vi "Send Receive Parse.vi"(8 "error in":errorcluster, 10 "Delay between send and receive [ms]":i32=100, 11 "<JSON>":string="{  \n    \"command\": \"ccd_discover\",\n    \"parameters\":{\n        \"index\": 0\n    }\n}") -> (0 "error out":errorcluster, 2 "ID":i32, 3 "results-JSON string":string)   [LabVIEW 2023, in "GenericDevice.lvclass"]
doc: "Wrapper around the send and receive calls."
uses:
  GenericDevice.lvclass
  Communicator/Communicator.lvclass
  DeviceManager/DeviceManager.lvlib
  <vilib>/JDP Science/JSONtext/JSONtext.lvlib
panel:
  # "Connector Pane"
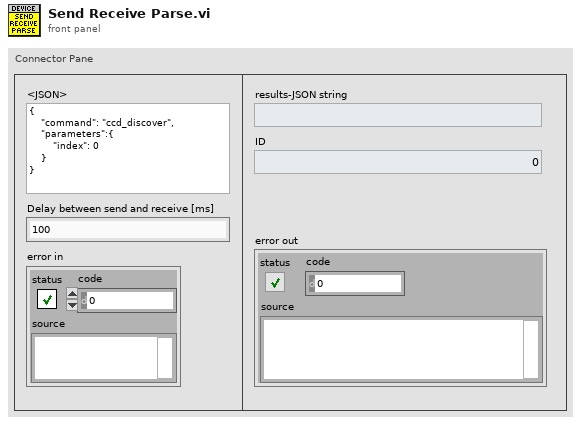
[diagram p1: front panel]
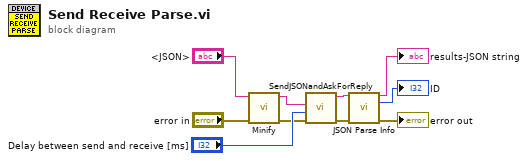
[diagram p0: block diagram]
diagram:
  n1 = call <vilib>:"Minify.vi"("error in (no error)"="error in", "JSON"="<JSON>") -> ("error out"=w3:errorcluster, "<JSON>"=w1:string)  [unwired: 7 in, 1 out]
  n2 = call "SendJSONandAskForReply.vi"("error in"=w3, "Delay between send and receive [ms]"="Delay between send and receive [ms]", "JSON to be sent"=w1) -> ("error out"=w5:errorcluster, "JSON reply"=w6:string)  [unwired: 6 in, 1 out]
  n3 = call "JSON Parse Info.vi"("JSON"=w6, "error in (no error)"=w5) -> ("results-JSON"=→"results-JSON string":string, "ID"=→"ID":i32, "error out"=→"error out":errorcluster)  [unwired: 11 in]
